vi "Initialize Global.vi"(8 "error in (no error)":errorcluster, 11 "UI Parameters":T1) -> (0 "error out":errorcluster)   [LabVIEW 2019, in "GaitDAQ UI.lvlib"]
uses:
  GaitDAQ UI.lvlib
  UI Parameters.ctl
  UI Refnums.ctl
  <userlib>/JUL/Event Message Module/Event Message Library/Event Message.lvlib
panel:
  # "Input"
  # "Output"
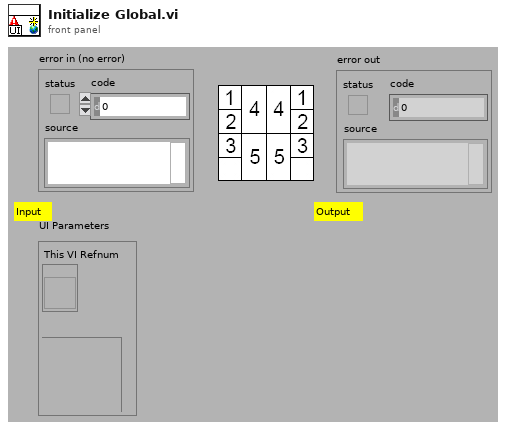
[diagram p1: front panel]
types:
  T1 = typedef "GaitDAQ UI.lvlib/UI Parameters.ctl" = cluster{"This VI Refnum":refnum<vi>, "UI Refnums":T2}
  T2 = typedef "GaitDAQ UI.lvlib/UI Refnums.ctl" = cluster{"Exit Refnum":refnum<vi>, "Camera Open or Close":refnum<vi>, "Camera Discover":refnum<vi>, "Camera":refnum<vi>, "Log or Unlog":refnum<vi>, "COM Open or Close":refnum<vi>, "COM Port":refnum<vi>, "Play or Pause":refnum<vi>, "Foot Image":refnum<vi>, "Data Folder":refnum<vi>, "Folder":refnum<vi>, "Data Path":refnum<vi>, "Load":refnum<vi>, "Stop":refnum<vi>, "Acquire or Review":refnum<vi>, "Slide":refnum<vi>}
  T3 = typedef "Event Message.lvlib/Event.ctl" = refnum<user-event>
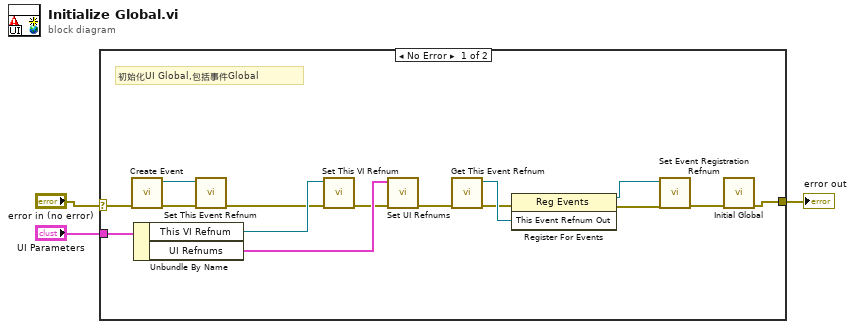
[diagram p0: block diagram]
diagram:
  n1 = case shown="No Error" "error in (no error)" {
    selector: "error in (no error)" -> [w17 w19]
    tunnel: [w4 w19] -> w2
    tunnel: "UI Parameters" -> [w10 _]
    frame No Error {
      # "初始化UI Global,包括事件Global"
      n2 = call <userlib>:"Create Event.vi"("error in (no error)"=w17) -> ("error out"=w16:errorcluster, "Event Out"=w18:T3)  [unwired: 9 in]
      n3 = Unbundle By Name(w10) -> ("This VI Refnum"=w8:refnum<vi>, "UI Refnums"=w9:T2)
      n4 = call "Set This Event Refnum.vi"("error in (no error)"=w16, "This Event Refnum In"=w18) -> ("error out"=w7:errorcluster)  [unwired: 9 in]
      n5 = call "Set This VI Refnum.vi"("error in (no error)"=w7, "This VI Refnum In"=w8) -> ("error out"=w6:errorcluster)  [unwired: 9 in]
      n6 = call "Set UI Refnums.vi"("error in (no error)"=w6, "Button 0 Refnum"=w9) -> ("error out"=w11:errorcluster)  [unwired: 9 in]
      n7 = call "Get This Event Refnum.vi"("error in (no error)"=w11) -> ("error out"=w14:errorcluster, "This Event Refnum Out"=w15:T3)  [unwired: 9 in]
      n8 = register-events(error in=w14, w15) -> (reference out=w12:refnum<event-registration>, error out=w13:errorcluster)  [unwired: 1 in]
      n9 = call "Set Event Registration Refnum.vi"("error in (no error)"=w13, "Event Registration Refnum in"=w12) -> ("error out"=w5:errorcluster)  [unwired: 9 in]
      n10 = call "Initial Global.vi"("error in (no error)"=w5) -> ("error out"=w4:errorcluster)  [unwired: 10 in]
    }
    frame Error {
    }
  }
  "error out" <- w2
